vi "SVI_ConvertStringBufferAndBuildGraphs.vi"(8 "Graphs In":T1, 10 "Time Step (ms)":i32, 11 "buffer":string) -> (0 "Graphs Out":T1, 3 "Current Values":T2)   [LabVIEW 2014]
panel:
  out "PD vs Time (s)":cluster{"Array":dbl[], "Array":dbl[]}
  out "PD vs Fine Temp Out":cluster{"Array":dbl[], "Array":dbl[]}
  out "Coarse Temp vs Time Out":cluster{"Array":dbl[], "Array":dbl[]}
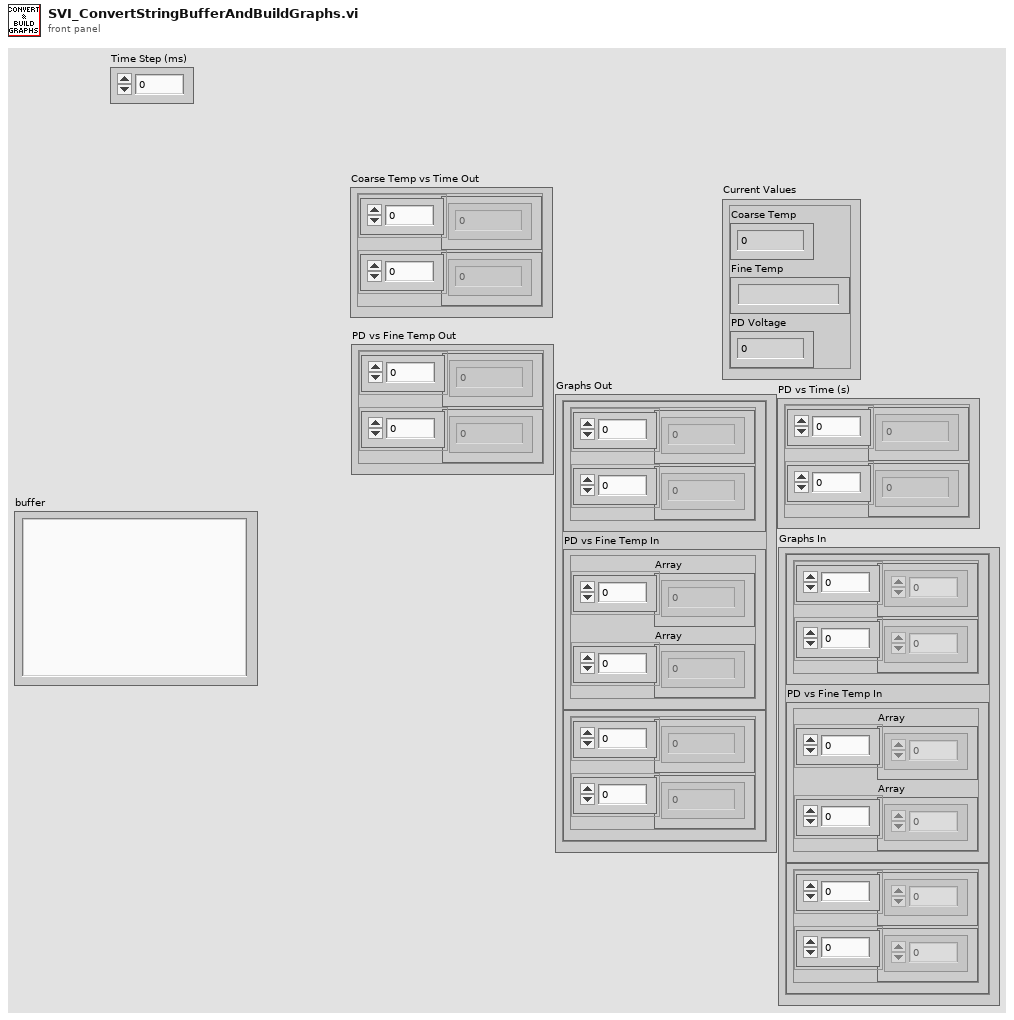
[diagram p1: front panel]
types:
  T1 = cluster{"Cluster":cluster{"Array":dbl[], "Array":dbl[]}, "PD vs Fine Temp In":cluster{"Array":dbl[], "Array":dbl[]}, "Cluster":cluster{"Array":dbl[], "Array":dbl[]}}
  T2 = cluster{"Coarse Temp":dbl, "Fine Temp":string, "PD Voltage":dbl}
  T3 = cluster{cluster{dbl[], dbl[]}, "PD vs Fine Temp In":cluster{"Array":dbl[], "Array":dbl[]}, cluster{dbl[], dbl[]}}
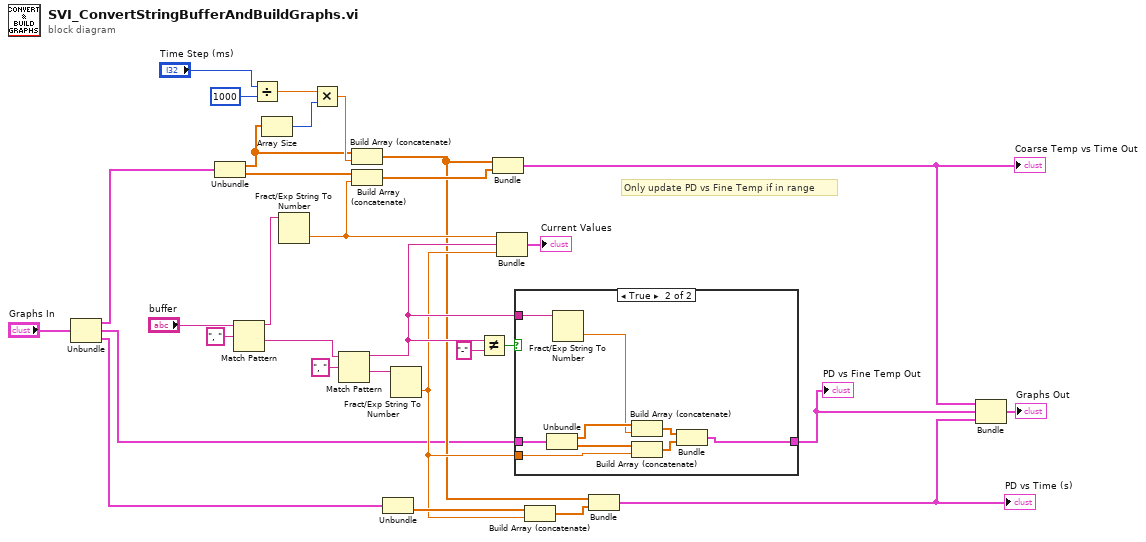
[diagram p0: block diagram]
diagram:
  # "Only update PD vs Fine Temp if in range"
  n1 = Unbundle("Graphs In") -> ("Cluster"=w1:cluster{"Array":dbl[], "Array":dbl[]}, "PD vs Fine Temp In"=w2:cluster{"Array":dbl[], "Array":dbl[]}, "Cluster"=w3:cluster{"Array":dbl[], "Array":dbl[]})
  n2 = Unbundle(w1) -> ("Array"=w14:dbl[], "Array"=w20:dbl[])
  n3 = Match Pattern(string="buffer", regular expression=", ") -> (before substring=w27:string, after substring=w28:string)  [unwired: 1 in, 2 out]
  n4 = Divide(x="Time Step (ms)", y=1000) -> (x/y=w23:dbl)
  n5 = Array Size(array=w14) -> (size(s)=w13:i32)
  n6 = Fract/Exp String To Number(string=w27) -> (number=w18:dbl)  [unwired: 3 in, 1 out]
  n7 = Multiply(x=w23, y=w13) -> (x*y=w21:dbl)
  n8 = Match Pattern(string=w28, regular expression=", ") -> (before substring=w16:string, after substring=w15:string)  [unwired: 1 in, 2 out]
  n9 = Build Array (concatenate)(w14, w21) -> (w7:dbl[])
  n10 = Build Array (concatenate)(w20, w18) -> (w19:dbl[])
  n11 = Unbundle(w3) -> ("Array"=w10:dbl[])  [unwired: 1 out]
  n12 = Fract/Exp String To Number(string=w15) -> (number=w9:dbl)  [unwired: 3 in, 1 out]
  n13 = Not Equal?(x=w16, y="-") -> (x != y?=w25:bool)
  n14 = Bundle(w7, w19) -> (w12:cluster{dbl[], dbl[]})  [unwired: 1 in]
  "Coarse Temp vs Time Out" <- w12
  n15 = Bundle(w18, "buffer"=w16, w9) -> (→"Current Values":cluster{dbl, "buffer":string, dbl})  [unwired: 1 in]
  n16 = case shown="True" w25 {
    tunnel: w16 -> [_ w41]
    tunnel: w2 -> [w32 w37]
    tunnel: [w32 w33] -> w11
    tunnel: w9 -> [_ w34]
    frame False {
    }
    frame True {
      n17 = Unbundle(w37) -> ("Array"=w36:dbl[], "Array"=w38:dbl[])
      n18 = Fract/Exp String To Number(string=w41) -> (number=w35:dbl)  [unwired: 3 in, 1 out]
      n19 = Build Array (concatenate)(w36, w35) -> (w39:dbl[])
      n20 = Build Array (concatenate)(w38, w34) -> (w40:dbl[])
      n21 = Bundle(w39, w40) -> (w33:cluster{dbl[], dbl[]})  [unwired: 1 in]
    }
  }
  "PD vs Fine Temp Out" <- w11
  n22 = Build Array (concatenate)(w10, w9) -> (w8:dbl[])
  n23 = Bundle(w7, w8) -> (w5:cluster{dbl[], dbl[]})  [unwired: 1 in]
  "PD vs Time (s)" <- w5
  n24 = Bundle(w12, "PD vs Fine Temp In"=w11, w5) -> (→"Graphs Out":T3)  [unwired: 1 in]
